vi "Continuous Gen 0-20mA Current.vi"() -> ()   [LabVIEW 2010]
doc: "I. Description:\nThis example demonstrates how to generate a single current value on one or more current output channels.\n\nII. Instructions for Running:\n1. Select the physical channel or channels which correspond to where your signal is to be generated.\n2. Enter the minimum and maximum current ranges, in amps (not milliamps).\n3. Enter a current value to generate in the data array. There should be one array value for each channel specified in the Physical Channels control. The values will be generated in the order that they appear in the Physical Channels control. \nNote: Just like the minimum and maximum current ranges, the data values to generate are in units of amps, not milliamps. \n\nIII. Block Diagram Steps:\n1. Create an analog output current channel.\n2. Call the Start VI to start the task.\n3. Use the Write VI to generate the data values on the\nspecified channels. Each element in the array contains\none current value for one channel specified in the \nPhysical Channels control.\n4. Call the Clear Task VI to clear the Task.\n5. Return any errors to the user in a dialog box.\n\nIV. I/O Connections Overview:\nThe SCXI-1124 can operate on either an external or internal current source. The only difference is in the signal connections. When using the internal current source, connect a load between the SUPPLY and ISINK terminals. When using an external current source, connect the source and load to the ISINK and GND terminals. In either case, be sure that the channel numbers of the terminals used match the channel numbers specified in the Physical Channels control.\n\nNote: When using an external current source, be careful to avoid creating an uncontrolled current loop. See the SCXI-1124 User's Manual for more information. \n\nThe NI 6238 and NI 6239 devices require external current sources. See the M Series User Manual for more information about signal connections to these devices.\n\nThe output current can be measured by connecting an ammeter in series with the current loop. Alternatively, the current can be measured by replacing the load with a resistor of known value. By measuring the voltage across the resistor and dividing by the resistance, the current through the resistor can be calculated (Ohm's law)."
uses:
  <vilib>/Utility/error.llb/DialogType.ctl
  <vilib>/DAQmx/write.llb/DAQmx Write (Analog 1D DBL NChan 1Samp).vi
  <vilib>/DAQmx/create/channels.llb/DAQmx Create Channel (AO-Current-Basic).vi
  <vilib>/daqmx/miscellaneous.llb/DAQmx Fill In Error Info.vi
panel:
  in  "Apply":bool
  in  "stop":bool
  in  "Physical Channels":tag="Dev1/ao0"
  in  "Data":dbl[](array[numeric])=[0.02] format="%0.3f"
  in  "Minimum Value":dbl format="%0.3f"
  in  "Maximum Value":dbl=0.02 format="%0.3f"
  # "For instructions, select Help>>Show Context Help"
  # "Channel Parameters"
  # "Current Values"
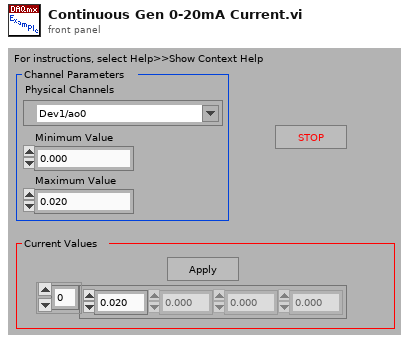
[diagram p1: front panel]
types:
  T1 = typedef "DialogType.ctl" = u16
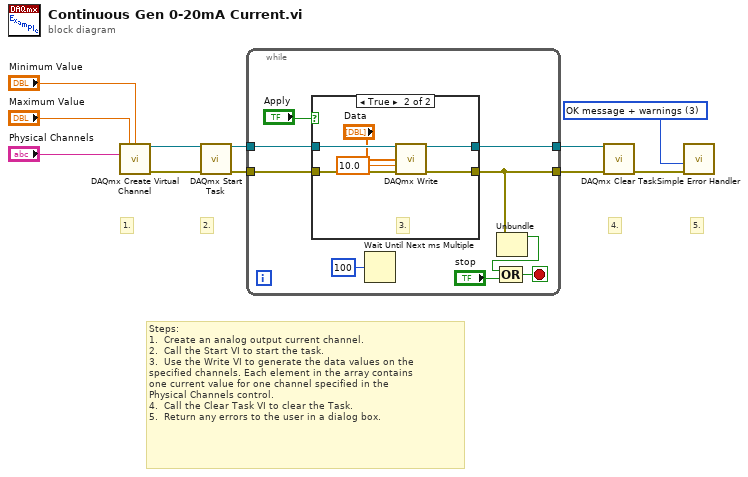
[diagram p0: block diagram]
diagram:
  w3 = T1 3 items=["no dialog", "OK message", "continue or stop message", "OK message + warnings", "continue/stop + warnings"] ("type of dialog (OK msg:1)")
  # "5."
  # "Steps: \n1.  Create an analog output current channel.\n2.  Call the Start VI to start the task.\n3.  Use the Write VI to generate the data values on the\nspecified channels. Each element in the array contains\none current value for one channel specified in the \nPhysical Channels control.\n4.  Call the Clear Task VI to clear the Task.\n5.  Return any errors to the user in a dialog box."
  # "1."
  # "2."
  # "4."
  n1 = call-poly <vilib>:"DAQmx Create Virtual Channel.vi"("maximum value"="Maximum Value", "minimum value"="Minimum Value", "physical channels"="Physical Channels") -> ("task out"=w9:refnum<k21>, "error out"=w8:errorcluster)  [unwired: 11 in]
  n2 = call <vilib>:"DAQmx Start Task.vi"("task/channels in"=w9, "error in"=w8) -> ("task out"=w7:refnum<k21>, "error out"=w6:errorcluster)  [unwired: 12 in]
  n3 = while {
    tunnel: w7 -> [w20]
    tunnel: w6 -> [w19]
    tunnel: [w18] -> w2
    tunnel: [w13] -> w1
    stop <- w14 stop-if-true
    n4 = case shown="True" "Apply" {
      tunnel: w20 -> [w21 w28]
      tunnel: w19 -> [w22 w27]
      tunnel: [w21 w24] -> w18
      tunnel: [w22 w23] -> w13
      frame False {
      }
      frame True {
        # "3."
        n5 = call-poly <vilib>:"DAQmx Write.vi"("task/channels in"=w28, "data"="Data", "timeout"=10.0, "error in"=w27) -> ("task out"=w24:refnum<k21>, "error out"=w23:errorcluster)  [unwired: 9 in, 1 out]
      }
    }
    n6 = Wait Until Next ms Multiple(millisecond multiple=u32 100) -> ()  [unwired: 1 out]
    n7 = Unbundle(w13) -> ("status"=w12:bool)  [unwired: 2 out]
    n8 = Compound Arithmetic op=OR(w12, "stop") -> (w14:bool)
  }
  n9 = call <vilib>:"DAQmx Clear Task.vi"("task in"=w2, "error in"=w1) -> ("error out"=w5:errorcluster)  [unwired: 13 in]
  n10 = call <vilib>:"Simple Error Handler.vi"("type of dialog (OK msg:1)"=w3, "error in (no error)"=w5) -> ()  [unwired: 3 in, 5 out]
